vi "NI USB-6218数据采集软件V12.vi"() -> ()   [LabVIEW 2024]
doc: "该范例演示了如何使用DAQmx设备连续采集带缓冲的电流信号。\n\n关于如何连接信号至DAQ设备，请查看设备文档。"
uses:
  <vilib>/DAQmx/read.llb/DAQmx Read (Analog 1D Wfm NChan NSamp).vi
  <vilib>/Analysis/baseanly.llb/Mean (DBL).vi
  <vilib>/Analysis/5stat.llb/RMS (DBL).vi
  <vilib>/DAQmx/create/channels.llb/DAQmx Create Channel (AI-Voltage-Basic).vi
  <vilib>/DAQmx/configure/timing.llb/DAQmx Timing (Sample Clock).vi
  <vilib>/Utility/file.llb/Write Delimited Spreadsheet (string).vi
  <vilib>/DAQmx/miscellaneous.llb/DAQmx Fill In Error Info.vi
  <vilib>/Utility/file.llb/Write Delimited Spreadsheet (DBL).vi
  <vilib>/Analysis/NI_AALBase.lvlib
  <vilib>/Analysis/NI_AALPro.lvlib
panel:
  in  "csv文件夹存储路径":path=path "C:/data/data.csv"
  in  "Manual Trig":bool
  in  "通信端口":u16=12345
  out "Auto Trig":bool
  out "Exit":bool
  in  "退出程序":bool
  out "位移均值曲线":waveform(dbl)(graph)
  out "校零参数":dbl[](array[numeric])
  in  "校零":bool
  out "加速度":waveform(dbl)[](graph)
  out "stop?":bool
  in  "程序运行时长(s)":dbl=30.0
  in  "风速仪换算-斜率":dbl=1.0
  in  "风速仪换算-截距":dbl
  in  "单点压力通道":tag="Dev4/ai6"
  out "位移":waveform(dbl)[](graph)
  out "风速仪":waveform(dbl)[](graph)
  out "压力":waveform(dbl)(graph)
  in  "位移换算-截距":dbl
  in  "位移换算-斜率":dbl=-20.0
  in  "风速仪通道":tag="Dev4/ai22, Dev4/ai30, Dev4/ai23, Dev4/ai31"
  in  "压力换算-截距":dbl
  in  "压力换算-斜率":dbl=1.0
  in  "位移通道":tag="Dev4/ai17:20"
  in  "停止":bool
  out "测力天平":waveform(dbl)[](graph)
  in  "每次循环采样数":i32=250
  in  "采样率":dbl=500.0
  in  "测力天平换算-斜率":dbl=1.0
  in  "测力天平换算-截距":dbl
  in  "测力天平通道":tag="Dev4/ai0:5"
  # "测力天平数据"
  # "风速仪数据"
  # "通道设置"
  # "加速度数据"
  # "位移数据"
  # "位移均值数据"
  # "压力数据"
  # "定时设置"
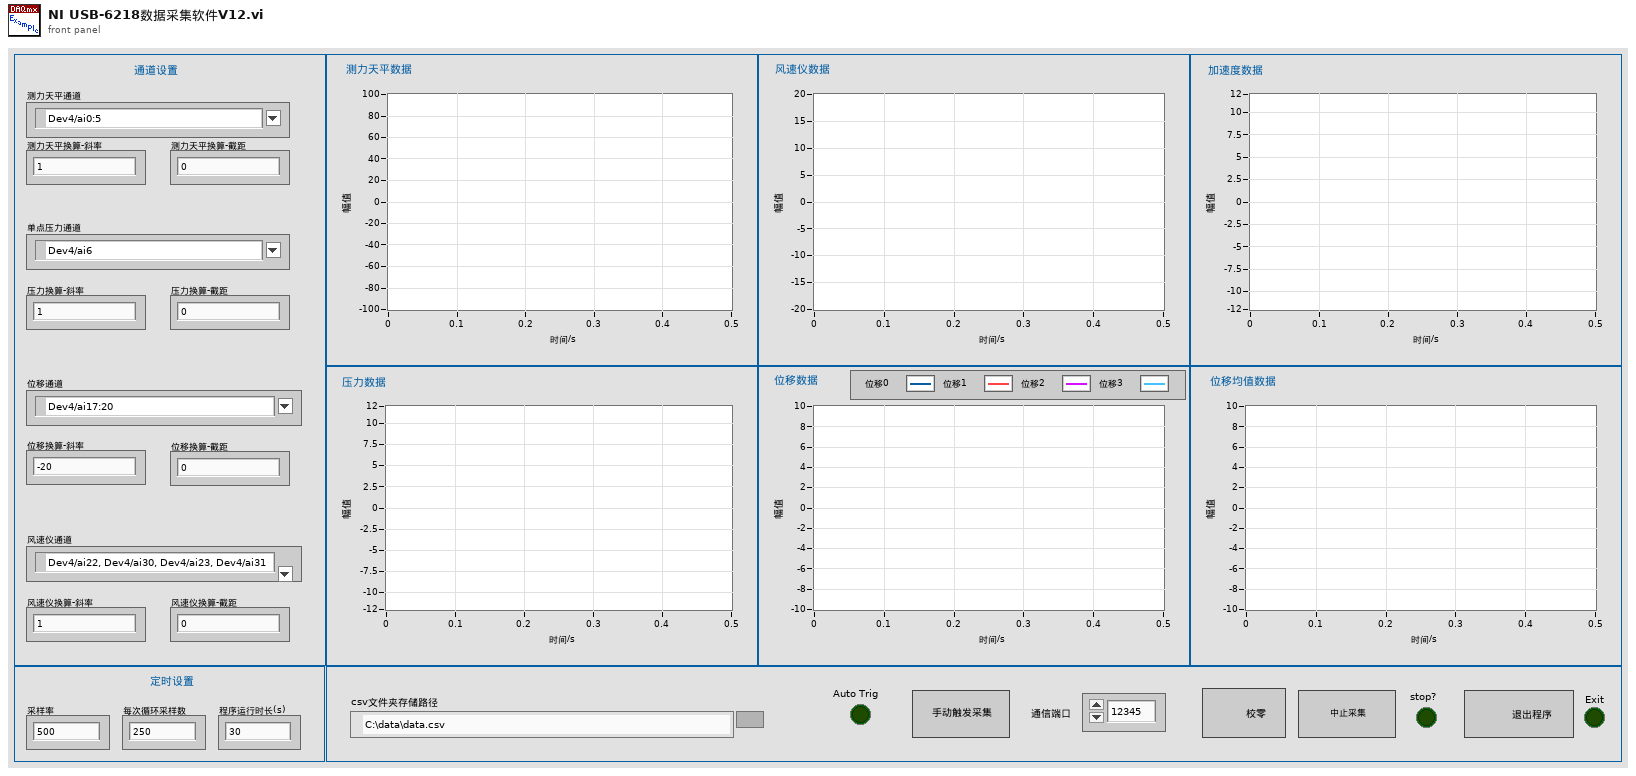
[diagram p1: front panel]
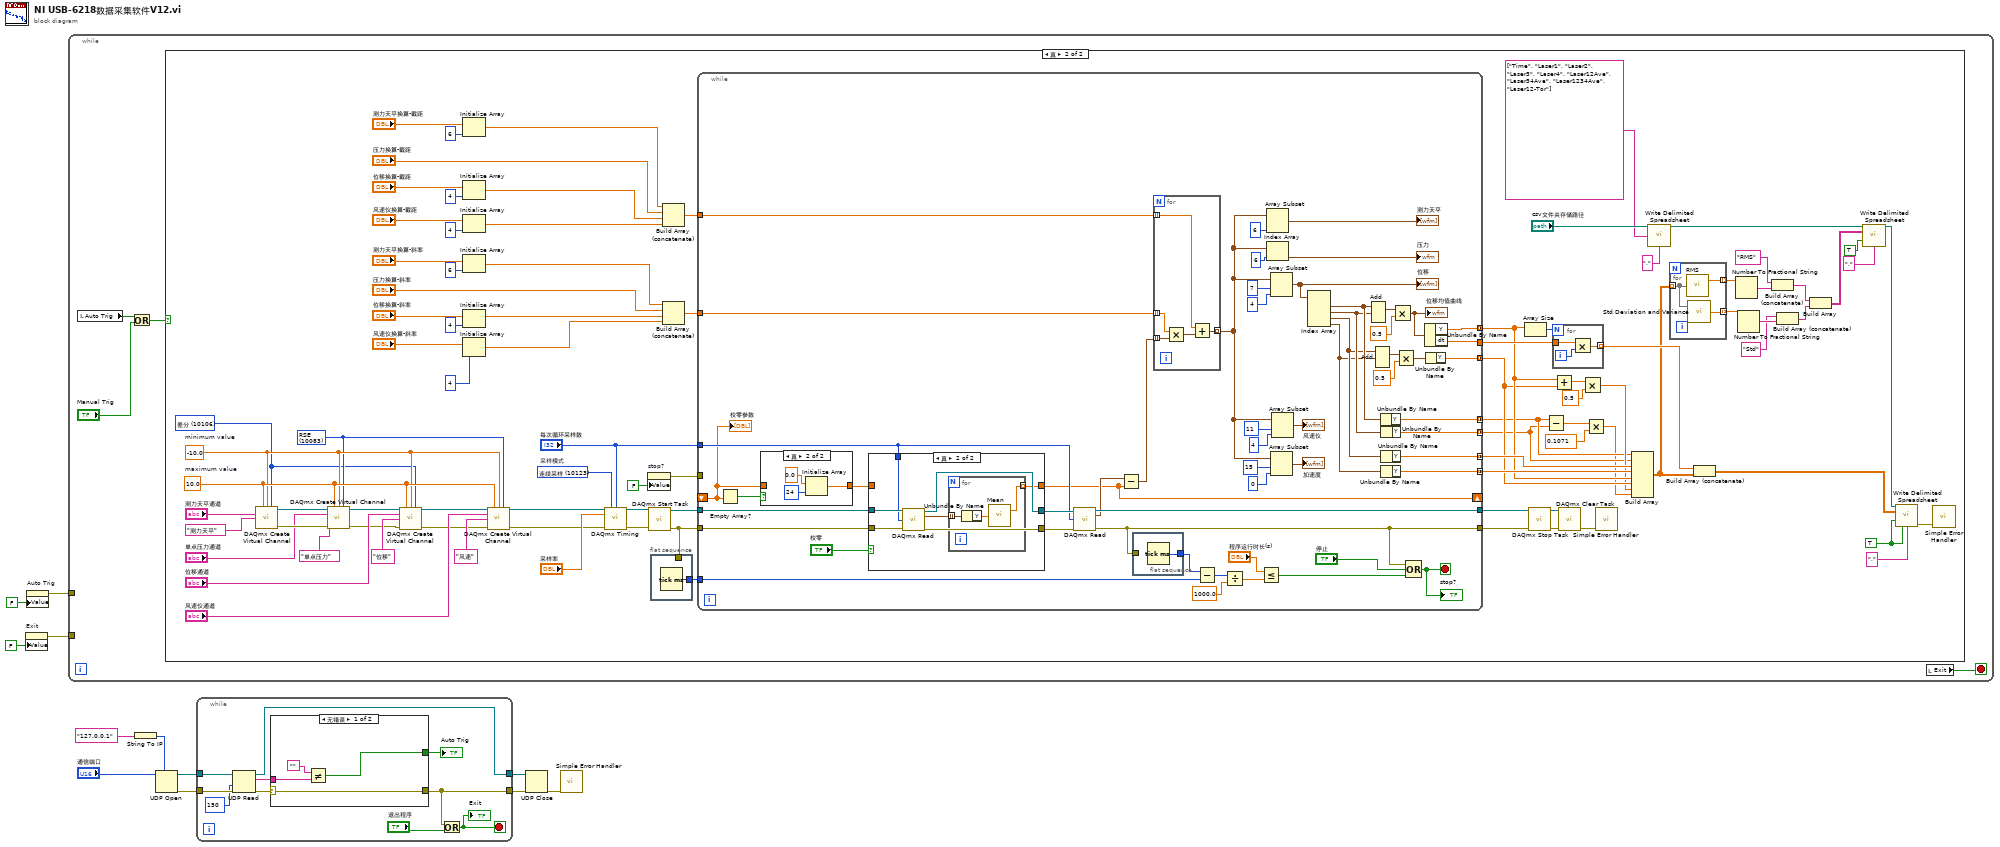
[diagram p0: block diagram]
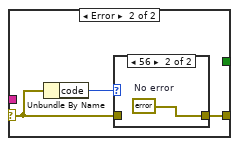
[diagram p2: hidden frame]
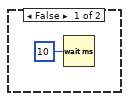
[diagram p4: hidden frame]
diagram:
  n1 = property on="Exit" class="Bool (严格)"("Value"=FALSE ("Exit")) -> (error out=w6:errorcluster)  [unwired: 2 in, 1 out]
  n2 = property on="Auto Trig" class="Bool (严格)"("Value"=FALSE ("Trig")) -> (error out=w4:errorcluster)  [unwired: 2 in, 1 out]
  n3 = while {
    tunnel: w6 -> [_]
    tunnel: w4 -> [_]
    stop <- w16 stop-if-true
    n4 = local read "Auto Trig"() -> (w14:bool)
    n5 = Or(x=w14, y="Manual Trig") -> (x .or. y?=w15:bool)
    n6 = case shown="真" w15 {
      frame False {
        n7 = Wait (ms)(milliseconds to wait=u32 10) -> ()  [unwired: 1 out]
      }
      frame True {
        w55 = TRUE ("transpose? (no:F)")
        w69 = 10083 items=["默认"=-1, "RSE"=10083, "NRSE"=10078, "差分"=10106, "伪差分"=12529] ("input terminal configuration")
        w64 = 10106 items=["默认"=-1, "RSE"=10083, "NRSE"=10078, "差分"=10106, "伪差分"=12529] ("input terminal configuration")
        w71 = 10.0  # maximum value
        w70 = -10.0  # minimum value
        w108 = 10123 items=["有限采样"=10178, "连续采样"=10123, "硬件定时单点"=12522]  # 采样模式
        n8 = call-poly <vilib>:"DAQmx Create Virtual Channel.vi"("maximum value"=w71, "minimum value"=w70, "input terminal configuration"=w64, "physical channels"="测力天平通道", "name to assign"="测力天平") -> ("task out"=w92:refnum<k21>, "error out"=w90:errorcluster)  [unwired: 9 in]
        n9 = call-poly <vilib>:"DAQmx Create Virtual Channel.vi"("task in"=w92, "maximum value"=w71, "minimum value"=w70, "input terminal configuration"=w69, "physical channels"="单点压力通道", "name to assign"="单点压力", "error in"=w90) -> ("task out"=w91:refnum<k21>, "error out"=w89:errorcluster)  [unwired: 7 in]
        n10 = call-poly <vilib>:"DAQmx Create Virtual Channel.vi"("task in"=w91, "maximum value"=w71, "minimum value"=w70, "input terminal configuration"=w64, "physical channels"="位移通道", "name to assign"="位移", "error in"=w89) -> ("task out"=w100:refnum<k21>, "error out"=w95:errorcluster)  [unwired: 7 in]
        n11 = Initialize Array("测力天平换算-截距", 6 ("维数大小")) -> (w83:dbl[])
        n12 = Initialize Array("位移换算-截距", 4 ("维数大小")) -> (w34:dbl[])
        n13 = Initialize Array("风速仪换算-截距", 4 ("维数大小")) -> (w76:dbl[])
        n14 = Initialize Array("测力天平换算-斜率", 6 ("维数大小")) -> (w79:dbl[])
        n15 = Initialize Array("位移换算-斜率", 4 ("维数大小")) -> (w31:dbl[])
        n16 = Initialize Array("风速仪换算-斜率", 4 ("维数大小")) -> (w73:dbl[])
        n17 = call-poly <vilib>:"DAQmx Create Virtual Channel.vi"("task in"=w100, "maximum value"=w71, "minimum value"=w70, "input terminal configuration"=w69, "physical channels"="风速仪通道", "name to assign"="风速", "error in"=w95) -> ("task out"=w68:refnum<k21>, "error out"=w67:errorcluster)  [unwired: 7 in]
        n18 = call-poly <vilib>:"DAQmx Timing.vi"("task/channels in"=w68, "sample mode"=w108, "samples per channel"="每次循环采样数", "rate"="采样率", "error in"=w67) -> ("task out"=w110:refnum<k21>, "error out"=w109:errorcluster)  [unwired: 9 in]
        n19 = property on="stop?" class="Bool (严格)"("Value"=FALSE ("stop?")) -> (error out=w61:errorcluster)  [unwired: 2 in, 1 out]
        n20 = call <vilib>:"DAQmx Start Task.vi"("task/channels in"=w110, "error in"=w109) -> ("task out"=w66:refnum<k21>, "error out"=w63:errorcluster)  [unwired: 12 in]
        n21 = flat-sequence {
          tunnel: [w117] -> w72
          tunnel: w63 -> [_]
          frame #0 {
            n22 = Tick Count (ms)() -> (millisecond timer value=w117:u32)
          }
        }
        n23 = Build Array (concatenate)(w83, "压力换算-截距", w34, w76) -> (w94:dbl[])
        n24 = Build Array (concatenate)(w79, "压力换算-斜率", w31, w73) -> (w93:dbl[])
        n25 = while {
          tunnel: w66 -> [w146]
          tunnel: w63 -> [w144]
          tunnel: [w136] -> w104
          tunnel: [w172] -> w105
          tunnel: "每次循环采样数" -> [w142]
          tunnel: w94 -> [w169]
          tunnel: w93 -> [w170]
          tunnel: w72 -> [w159]
          shift-right: [w141] -> _
          shift-left: _ -> [w137]
          tunnel: [w131] -> w28 mode=concatenating
          tunnel: [w130] -> w58
          tunnel: w61 -> [_]
          tunnel: [w127] -> w24 mode=concatenating
          tunnel: [w126] -> w23 mode=concatenating
          tunnel: [w125] -> w30 mode=concatenating
          tunnel: [w124] -> w29 mode=concatenating
          tunnel: [w118] -> w27 mode=concatenating
          stop <- w173 stop-if-true
          n26 = Empty Array?(array=w137) -> (empty?=w139:bool)
          n27 = case shown="真" w139 {
            tunnel: [w175 w176] -> w138
            tunnel: w137 -> [w175 _]
            frame False {
            }
            frame True {
              n28 = Initialize Array(0.0, 24 ("维数大小")) -> (w176:dbl[])
            }
          }
          n29 = case shown="真" "校零" {
            tunnel: w146 -> [w181 w188]
            tunnel: [w181 w187] -> w145
            tunnel: w144 -> [w180 w186]
            tunnel: [w180 w185] -> w143
            tunnel: w142 -> [_ w184]
            tunnel: [w179 w182] -> w141
            tunnel: w138 -> [w179 _]
            frame False {
            }
            frame True {
              n30 = call-poly <vilib>:"DAQmx Read.vi"("task/channels in"=w188, "number of samples per channel"=w184, "error in"=w186) -> ("task out"=w187:refnum<k21>, "data"=w183:waveform(dbl)[], "error out"=w185:errorcluster)  [unwired: 10 in]
              n31 = for {
                tunnel: w183 -> [w191] mode=indexing
                tunnel: [w189] -> w182 mode=indexing
                n32 = Unbundle By Name(w191) -> ("Y"=w190:dbl[])
                n33 = call-poly <vilib>:"Mean.vi"("X"=w190) -> ("mean"=w189:dbl)  [unwired: 1 out]
              }
            }
          }
          n34 = call-poly <vilib>:"DAQmx Read.vi"("task/channels in"=w145, "number of samples per channel"=w142, "error in"=w143) -> ("task out"=w172:refnum<k21>, "data"=w148:waveform(dbl)[], "error out"=w136:errorcluster)  [unwired: 10 in]
          n35 = Subtract(x=w148, y=w141) -> (x-y=w147:waveform(dbl)[])
          n36 = flat-sequence {
            tunnel: [w174] -> w160
            tunnel: w136 -> [_]
            frame #0 {
              n37 = Tick Count (ms)() -> (millisecond timer value=w174:u32)
            }
          }
          n38 = for {
            tunnel: w147 -> [w196] mode=indexing
            tunnel: w170 -> [w195] mode=indexing
            tunnel: w169 -> [w193] mode=indexing
            tunnel: [w192] -> w150 mode=indexing
            n39 = Multiply(x=w195, y=w196) -> (x*y=w194:waveform(dbl))
            n40 = Add(x=w193, y=w194) -> (x+y=w192:waveform(dbl))
          }
          n41 = Subtract(x=w160, y=w159) -> (x-y=w158:u32)
          n42 = Divide(x=w158, y=1000.0) -> (x/y=w155:dbl)
          n43 = Less Or Equal?(x="程序运行时长(s)", y=w155) -> (x <= y?=w154:bool)
          n44 = Array Subset(array=w150, length=6 ("长度")) -> (→"测力天平":waveform(dbl)[])  [unwired: 1 in]
          n45 = Index Array(array=w150, index=6 ("长度")) -> (element=→"压力":waveform(dbl))
          n46 = Array Subset(array=w150, index=7 ("索引"), length=4 ("索引")) -> (w133:waveform(dbl)[])
          "位移" <- w133
          n47 = Array Subset(array=w150, index=15 ("索引"), length=0 ("索引")) -> (→"加速度":waveform(dbl)[])
          n48 = Array Subset(array=w150, index=11 ("索引"), length=4 ("索引")) -> (→"风速仪":waveform(dbl)[])
          n49 = Index Array(array=w133) -> (element #1=w129:waveform(dbl), element #2=w128:waveform(dbl), element #3=w121:waveform(dbl), element #4=w120:waveform(dbl))  [unwired: 4 in]
          n50 = Add(1:w128, 2:w129) -> (0:w135:waveform(dbl))  [unwired: 1 in, 1 out]
          n51 = Add(1:w120, 2:w121) -> (0:w122:waveform(dbl))  [unwired: 1 in, 1 out]
          n52 = Unbundle By Name(w129) -> ("Y"=w127:dbl[])
          n53 = Unbundle By Name(w128) -> ("Y"=w126:dbl[])
          n54 = Unbundle By Name(w121) -> ("Y"=w125:dbl[])
          n55 = Unbundle By Name(w120) -> ("Y"=w124:dbl[])
          n56 = Multiply(x=w135, y=0.5) -> (x*y=w132:waveform(dbl))
          "位移均值曲线" <- w132
          n57 = Multiply(x=w122, y=0.5) -> (x*y=w119:waveform(dbl))
          n58 = Compound Arithmetic op=OR ("复合运算")(w136, "停止", w154) -> (w173:bool)
          "stop?" <- w173
          n59 = Unbundle By Name(w132) -> ("Y"=w131:dbl[], "dt"=w130:dbl)
          n60 = Unbundle By Name(w119) -> ("Y"=w118:dbl[])
          "校零参数" <- w137
        }
        n61 = Array Size(array=w28) -> (size(s)=w59:i32)
        n62 = call <vilib>:"DAQmx Stop Task.vi"("task/channels in"=w105, "error in"=w104) -> ("task out"=w103:refnum<k21>, "error out"=w102:errorcluster)  [unwired: 12 in]
        n63 = Subtract(x=w24, y=w23) -> (x-y=w21:dbl[])
        n64 = for {
          N: w59 -> [_]
          tunnel: w58 -> [w116]
          tunnel: [w114] -> w50 mode=indexing
          i -> [w115]
          n65 = Multiply(x=w116, y=w115) -> (x*y=w114:dbl)
        }
        n66 = Add(x=w28, y=w27) -> (x+y=w26:dbl[])
        n67 = call <vilib>:"DAQmx Clear Task.vi"("task in"=w103, "error in"=w102) -> ("error out"=w60:errorcluster)  [unwired: 13 in]
        n68 = Multiply(x=w26, y=0.5) -> (x*y=w25:dbl[])
        n69 = Multiply(x=w21, y=0.1071) -> (x*y=w19:dbl[])
        n70 = call <vilib>:"Simple Error Handler.vi"("error in (no error)"=w60) -> ()  [unwired: 4 in, 5 out]
        n71 = Build Array(w24, w23, w30, w29, w28, w27, w25, w19) -> (w48:dbl[][])
        n72 = call-poly <vilib>:"Write Delimited Spreadsheet.vi"("file path (dialog if empty)"="csv文件夹存储路径", "1D data"=string[] ["Time", "Laser1", "Laser2", "Laser3", "Laser4", "Laser12Ave", "Laser34Ave", "Laser1234Ave", "Laser12-Tor"], "delimiter (\\t)"="," ("delimiter (\\t)")) -> ("new file path (Not A Path if cancelled)"=w18:path)  [unwired: 11 in, 1 out]
        n73 = for {
          tunnel: w48 -> [w112] mode=indexing
          tunnel: [w113] -> w46 mode=indexing
          tunnel: [w111] -> w42 mode=indexing
          n74 = call-poly <vilib>:"RMS.vi"("X"=w112) -> ("rms value"=w113:dbl)  [unwired: 1 out]
          n75 = call <vilib>:"Std Deviation and Variance.vi"("X"=w112) -> ("standard deviation"=w111:dbl)  [unwired: 1 in, 2 out]
        }
        n76 = Build Array (concatenate)(w50, w48) -> (w49:dbl[][])
        n77 = Number To Fractional String(number=w46) -> (F-format string=w45:string[])  [unwired: 3 in]
        n78 = Number To Fractional String(number=w42) -> (F-format string=w41:string[])  [unwired: 3 in]
        n79 = Build Array (concatenate)("RMS", w45) -> (w40:string[])
        n80 = Build Array (concatenate)("Std", w41) -> (w39:string[])
        n81 = Build Array(w40, w39) -> (w37:string[][])
        n82 = call-poly <vilib>:"Write Delimited Spreadsheet.vi"("file path (dialog if empty)"=w18, "2D data"=w37, "append to file? (new file:F)"=TRUE, "delimiter (\\t)"="," ("delimiter (\\t)")) -> ("new file path (Not A Path if cancelled)"=w51:path)  [unwired: 10 in, 1 out]
        n83 = call-poly <vilib>:"Write Delimited Spreadsheet.vi"("file path (dialog if empty)"=w51, "2D data"=w49, "append to file? (new file:F)"=w55, "transpose? (no:F)"=w55, "delimiter (\\t)"="," ("delimiter (\\t)")) -> ("error out"=w56:errorcluster)  [unwired: 9 in, 1 out]
        n84 = call <vilib>:"Simple Error Handler.vi"("error in (no error)"=w56) -> ()  [unwired: 4 in, 5 out]
      }
    }
    n85 = local read "Exit"() -> (w16:bool)
  }
  n86 = String To IP(1:"127.0.0.1") -> (0:w1:u32)
  n87 = UDP Open(7:w1, 11:"通信端口") -> (port=w8:refnum<k16>, 0:w9:errorcluster)  [unwired: 3 in, 1 out]
  n88 = while {
    tunnel: w8 -> [w206]
    tunnel: [w198] -> w12
    tunnel: w9 -> [w203]
    tunnel: [w199] -> w10
    stop <- w204 stop-if-true
    n89 = UDP Read(connection ID=w206, timeout ms (25000)=150, 8:w203) -> (data out=w201:string, error out=w200:errorcluster, 3:w198:refnum<k16>)  [unwired: 3 out]
    n90 = case shown="无错误" w200 {
      selector: w200 -> [w210 w212]
      tunnel: w201 -> [w208 _]
      tunnel: [w210 w211] -> w199
      tunnel: [w207 _] -> w197
      frame No Error {
        n91 = Not Equal?(x="", y=w208) -> (x != y?=w207:bool)
      }
      frame Error {
        # "Sender did not send data. Ignore timeout error and keep waiting."
        n92 = Unbundle By Name(w212) -> ("code"=w213:i32)
        n93 = case shown="56" w213 {
          tunnel: w212 -> [w214 _]
          tunnel: [w214 w215] -> w211
          frame Default {
          }
          frame 56 {
            w215 = errorcluster {"status"=FALSE, "code"=0, "source"=""}  # No error
          }
        }
      }
    }
    "Auto Trig" <- w197
    n94 = Or(x=w199, y="退出程序") -> (x .or. y?=w204:bool)
    "Exit" <- w204
  }
  n95 = UDP Close(connection ID=w12, 8:w10) -> (error out=w11:errorcluster)  [unwired: 1 out]
  n96 = call <vilib>:"Simple Error Handler.vi"("error in (no error)"=w11) -> ()  [unwired: 1 in, 8 out]
